vi "Output Variants.vi"(6 "String Array":string[](array[string])=["str1", "str2", "str3"], 7 "Boolean Array":bool[](array[boolean])=[TRUE, FALSE, TRUE, FALSE], 8 "Numeric Array":dbl[](array[numeric])=[1.0, 2.0, 3.0] format="%0.2f", 9 "String":string="hello", 10 "Boolean":bool=TRUE, 11 "Numeric":u16=4) -> (0 "Numeric Array Variant":variant=variant(u8[] [1, 2, 3]), 1 "String Variant":variant=variant(string "hello"), 2 "Boolean Variant":variant=variant(bool TRUE), 3 "Numeric Variant":variant=variant(dbl 4.0), 4 "String Array Variant":variant=variant(string[] ["str1", "str2", "str3"]), 5 "Boolean Array Variant":variant=variant(bool[] [TRUE, FALSE, TRUE, FALSE]))   [LabVIEW 2012]
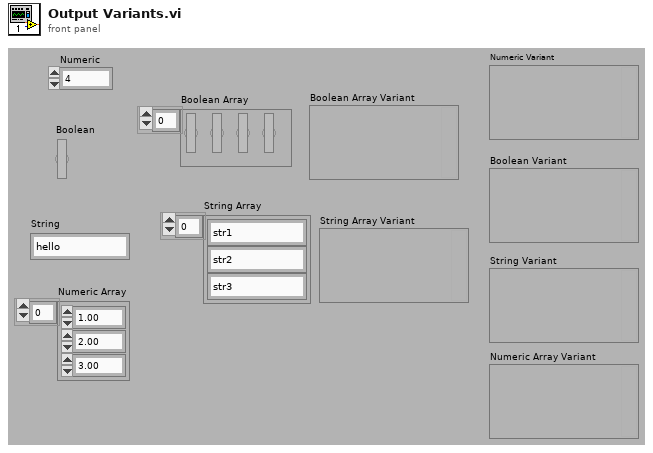
[diagram p1: front panel]
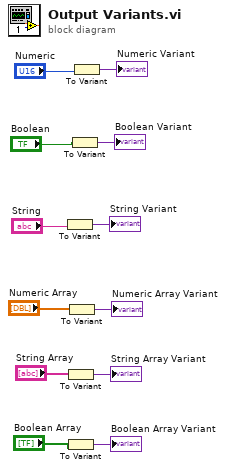
[diagram p0: block diagram]
diagram:
  n1 = To Variant(anything="String") -> (Variant=→"String Variant":variant)
  n2 = To Variant(anything="String Array") -> (Variant=→"String Array Variant":variant)
  n3 = To Variant(anything="Boolean Array") -> (Variant=→"Boolean Array Variant":variant)
  n4 = To Variant(anything="Numeric Array") -> (Variant=→"Numeric Array Variant":variant)
  n5 = To Variant(anything="Boolean") -> (Variant=→"Boolean Variant":variant)
  n6 = To Variant(anything="Numeric") -> (Variant=→"Numeric Variant":variant)
